vi "CRYListbox Editor.vi"(7 "In Check":bool[](array[boolean]), 8 "In Items":string[](array[string]), 9 "In Type":string) -> (1 "Out Check":bool[](array[boolean]), 2 "Out Items":string[](array[string]))   [LabVIEW 2013]
panel:
  out "Out Check 2":bool[](array[boolean])
  out "Out Items 2":string[](array[string])
  out "Unit":string
  out "Listbox_Unit":string
  in  "End":dbl format="%#.6p"
  in  "Begin":dbl format="%#.6p"
  in  "to":bool
  in  "Search Range":i32(listbox) caption="aa"
  in  "Cancel":bool
  in  "OK":bool
  in  "Remove":bool
  in  "Add":bool
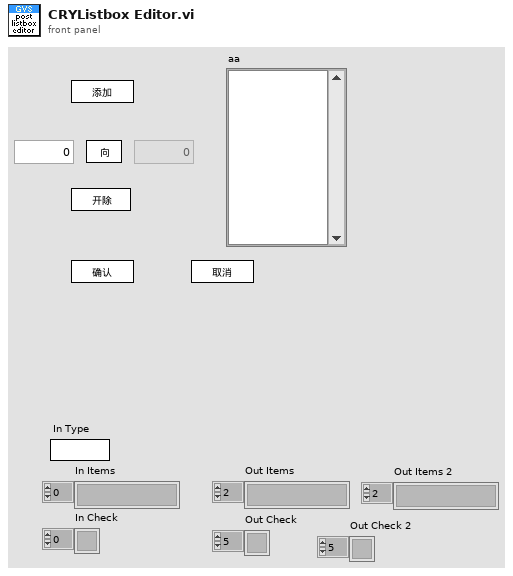
[diagram p1: front panel]
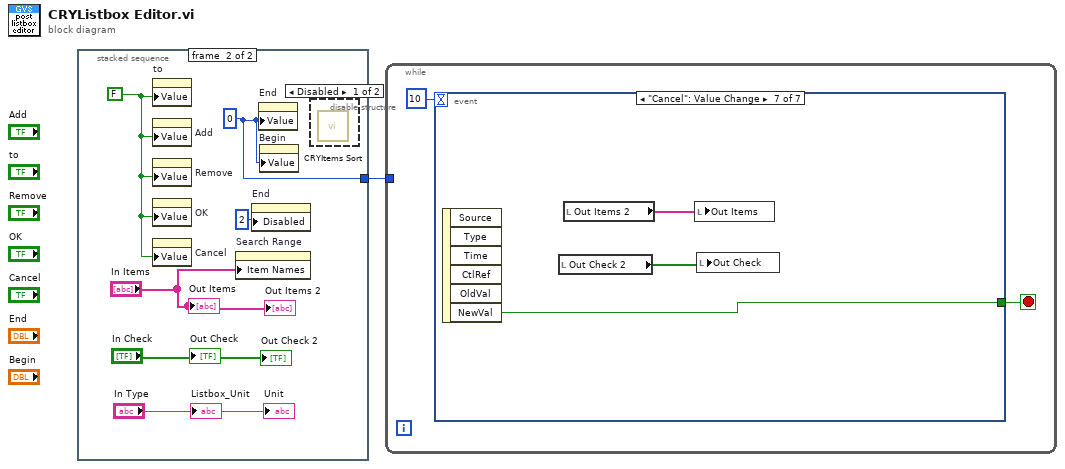
[diagram p0: block diagram]
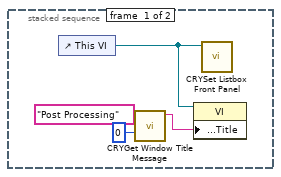
[diagram p2: hidden frame]
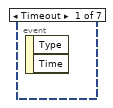
[diagram p4: hidden frame]
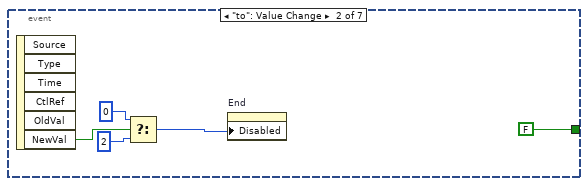
[diagram p5: hidden frame]
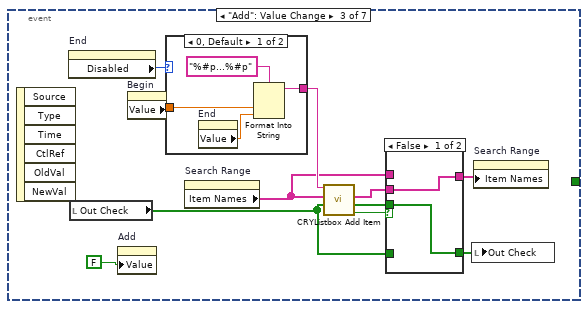
[diagram p6: hidden frame]
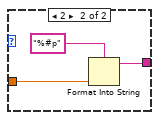
[diagram p8: hidden frame]
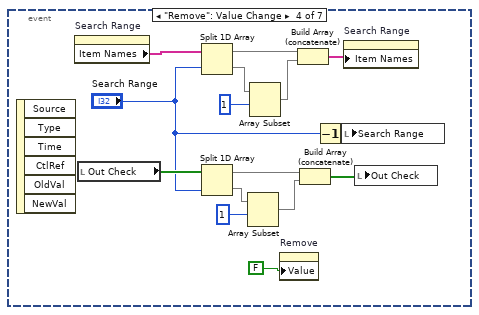
[diagram p9: hidden frame]
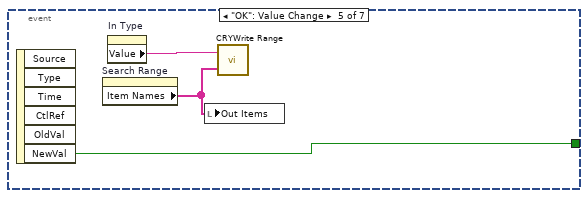
[diagram p10: hidden frame]
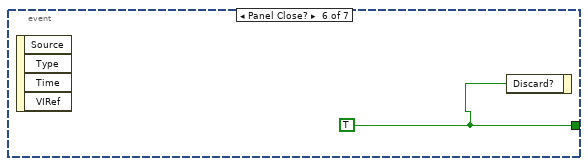
[diagram p11: hidden frame]
diagram:
  n1 = stacked-sequence {
    tunnel: [_ w8] -> w1
    frame #0 {
      n2 = control-ref of="This VI"() -> (w3:refnum<vi>)
      n3 = call "CRYGet Window Title Message.vi"("No"=0, "Kind"="Post Processing") -> ("Multibyte String"=w2:string)  [unwired: 4 in, 5 out]
      n4 = property class="VI"(reference=w3, "Front Panel.Title"=w2) -> ()  [unwired: 1 in, 2 out]
      n5 = call "CRYSet Listbox Front Panel.vi"("Vi Ref"=w3) -> ()  [unwired: 11 in]
    }
    frame #1 {
      w8 = 0 ("End")
      w10 = FALSE ("to")
      n6 = property on="to" class="Bool (strict)"("Value"=w10) -> ()  [unwired: 2 in, 2 out]
      n7 = property on="Add" class="Bool (strict)"("Value"=w10) -> ()  [unwired: 2 in, 2 out]
      n8 = property on="Remove" class="Bool (strict)"("Value"=w10) -> ()  [unwired: 2 in, 2 out]
      n9 = property on="OK" class="Bool (strict)"("Value"=w10) -> ()  [unwired: 2 in, 2 out]
      n10 = property on="Cancel" class="Bool (strict)"("Value"=w10) -> ()  [unwired: 2 in, 2 out]
      n11 = property on="Search Range" class="LstBox (strict)"("Item Names"="In Items") -> ()  [unwired: 2 in, 2 out]
      n12 = property on="End" class="DigNum (strict)"("Disabled"=u8 2) -> ()  [unwired: 2 in, 2 out]
      n13 = property on="End" class="DigNum (strict)"("Value"=w8) -> ()  [unwired: 2 in, 2 out]
      n14 = property on="Begin" class="DigNum (strict)"("Value"=w8) -> ()  [unwired: 2 in, 2 out]
      n15 = disable-structure shown="Disabled" {
        frame Disabled {
          n16 = call "CRYItems Sort.vi"() -> ()  [unwired: 3 in, 9 out]
        }
        frame Enabled {
        }
      }
      "Listbox_Unit" <- "In Type"
      "Unit" <- "In Type"
      "Out Items" <- "In Items"
      "Out Check" <- "In Check"
      "Out Items 2" <- "In Items"
      "Out Check 2" <- "In Check"
    }
  }
  n17 = while {
    tunnel: w1 -> [_]
    stop <- w12 stop-if-true
    n18 = event shown="[6] \"Cancel\": Value Change" {
      selector: _ -> [_ _ _ _ _ _ _]
      dyn-events: _ -> [_ _ _ _ _ _ _]
      timeout: 10 -> [_ _ _ _ _ _ _]
      tunnel: [_ FALSE ("NewVal") _ _ w56 w59 w62] -> w12
      event Timeout {
        n19 = event-data() -> ()  [unwired: 3 out]
      }
      event "to": Value Change {
        n20 = event-data() -> ("NewVal"=w18:bool)  [unwired: 6 out]
        n21 = Select(t=u8 0 ("Disabled"), s=w18, f=u8 2 ("Disabled")) -> (s? t:f=w15:u8)
        n22 = property on="End" class="DigNum (strict)"("Disabled"=w15) -> ()  [unwired: 2 in, 2 out]
      }
      event "Add": Value Change {
        n23 = event-data() -> ()  [unwired: 7 out]
        n24 = property on="End" class="DigNum (strict)"() -> ("Disabled"=w29:u8)  [unwired: 2 in, 2 out]
        n25 = local read "Out Check"() -> (w20:bool[])
        n26 = property on="Add" class="Bool (strict)"("Value"=FALSE ("Add")) -> ()  [unwired: 2 in, 2 out]
        n27 = property on="Begin" class="DigNum (strict)"() -> ("Value"=w28:dbl)  [unwired: 2 in, 2 out]
        n28 = case shown="0, Default" w29 {
          tunnel: w28 -> [w35 w39]
          tunnel: [w36 w38] -> w27
          frame 0, Default {
            n29 = property on="End" class="DigNum (strict)"() -> ("Value"=w34:dbl)  [unwired: 2 in, 2 out]
            n30 = Format Into String(format string="%#p...%#p", w35, w34) -> (resulting string=w36:string)  [unwired: 2 in, 1 out]
          }
          frame 2 {
            n31 = Format Into String(format string="%#p", w39) -> (resulting string=w38:string)  [unwired: 2 in, 1 out]
          }
        }
        n32 = property on="Search Range" class="LstBox (strict)"() -> ("Item Names"=w23:string[])  [unwired: 2 in, 2 out]
        n33 = call "CRYListbox Add Item.vi"("Check In"=w20, "Items In"=w23, "Candidate item In"=w27) -> ("Cancel operation Out"=w26:bool, "Check Out"=w22:bool[], "Items Out"=w24:string[])  [unwired: 6 out]
        n34 = case shown="False" w26 {
          tunnel: [w31 w33] -> w25
          tunnel: w24 -> [w31 _]
          tunnel: [w30 w32] -> w19
          tunnel: w20 -> [_ w32]
          tunnel: w23 -> [_ w33]
          tunnel: w22 -> [w30 _]
          frame False {
          }
          frame True {
          }
        }
        n35 = local write "Out Check"(w19) -> ()
        n36 = property on="Search Range" class="LstBox (strict)"("Item Names"=w25) -> ()  [unwired: 2 in, 2 out]
      }
      event "Remove": Value Change {
        n37 = event-data() -> ()  [unwired: 7 out]
        n38 = property on="Search Range" class="LstBox (strict)"() -> ("Item Names"=w51:string[])  [unwired: 2 in, 2 out]
        n39 = local read "Out Check"() -> (w47:bool[])
        n40 = Split 1D Array(array=w51, index="Search Range") -> (first subarray=w52:string[], second subarray=w50:string[])
        n41 = Split 1D Array(array=w47, index="Search Range") -> (first subarray=w46:bool[], second subarray=w45:bool[])
        n42 = Array Subset(array=w45, index=1) -> (w44:bool[])  [unwired: 1 in]
        n43 = Array Subset(array=w50, index=1 ("Array Index")) -> (w54:string[])  [unwired: 1 in]
        n44 = property on="Remove" class="Bool (strict)"("Value"=FALSE ("Remove")) -> ()  [unwired: 2 in, 2 out]
        n45 = Build Array (concatenate)(w52, w54) -> (w53:string[])
        n46 = Build Array (concatenate)(w46, w44) -> (w42:bool[])
        n47 = Decrement(x="Search Range") -> (x-1=w48:i32)
        n48 = local write "Search Range"(w48) -> ()
        n49 = property on="Search Range" class="LstBox (strict)"("Item Names"=w53) -> ()  [unwired: 2 in, 2 out]
        n50 = local write "Out Check"(w42) -> ()
      }
      event "OK": Value Change {
        n51 = event-data() -> ("NewVal"=w56:bool)  [unwired: 6 out]
        n52 = property on="Search Range" class="LstBox (strict)"() -> ("Item Names"=w57:string[])  [unwired: 2 in, 2 out]
        n53 = property on="In Type" class="Str"() -> ("Value"=w58:string)  [unwired: 2 in, 2 out]
        n54 = local write "Out Items"(w57) -> ()
        n55 = call "CRYWrite Range.vi"("In Items"=w57, "In Unit"=w58) -> ()  [unwired: 1 out]
      }
      event Panel Close? {
        w59 = TRUE ("NewVal")
        n56 = event-data() -> ()  [unwired: 5 out]
        n57 = event-data("Discard?"=w59) -> ()  [unwired: 1 in, 1 out]
      }
      event "Cancel": Value Change {
        n58 = event-data() -> ("NewVal"=w62:bool)  [unwired: 6 out]
        n59 = local read "Out Check 2"() -> (w60:bool[])
        n60 = local read "Out Items 2"() -> (w61:string[])
        n61 = local write "Out Items"(w61) -> ()
        n62 = local write "Out Check"(w60) -> ()
      }
    }
  }
